vi "Read Digital Port.vi"(8 "error in (no error)":errorcluster, 11 "Sim DIO in":refnum<class "Sim DIO.lvclass">) -> (0 "error out":errorcluster, 2 "Relay Mode":bool[](array[boolean]), 3 "Sim DIO out":refnum<class "Sim DIO.lvclass">)   [LabVIEW 2019, in "Concrete.lvlib" / "Sim DIO.lvclass"]
uses:
  Sim DIO.lvclass
  Harware Abstraction/DIO/DIO.lvclass
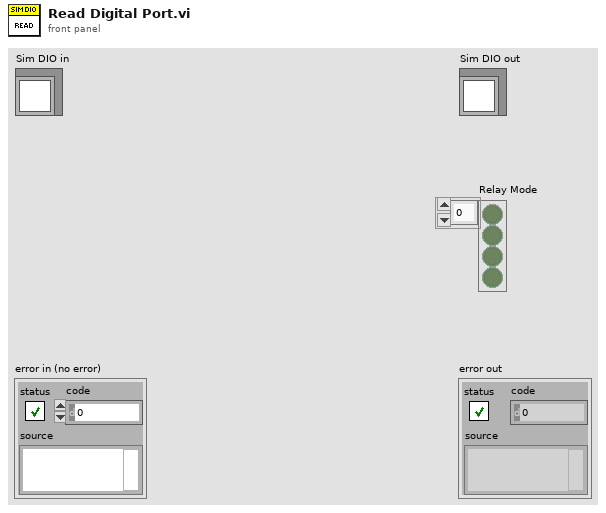
[diagram p1: front panel]
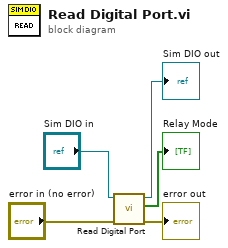
[diagram p0: block diagram]
diagram:
  n1 = call-parent "Read Digital Port.vi"("error in (no error)"="error in (no error)", "DIO in"="Sim DIO in") -> ("error out"=→"error out":errorcluster, "Relay Mode"=→"Relay Mode":bool[], "DIO out"=→"Sim DIO out":refnum<class "Sim DIO.lvclass">)  [unwired: 7 in]
